vi "UpdateList.vi"(8 "error in (no error)":errorcluster, 11 "Prooduct Actor in":refnum<class "Prooduct Actor.lvclass">) -> (0 "error out":errorcluster, 3 "Prooduct Actor out":refnum<class "Prooduct Actor.lvclass">)   [LabVIEW 2020, in "Prooduct Actor.lvlib" / "Prooduct Actor.lvclass"]
uses:
  Prooduct Actor.lvclass
  Controls/Language Enum.ctl
  Controls/Currency Enum.ctl
  Prooduct Actor.lvclass/Prooduct Actor.ctl
  Read Currency.vi
  Read Language.vi
  Read DBPath.vi
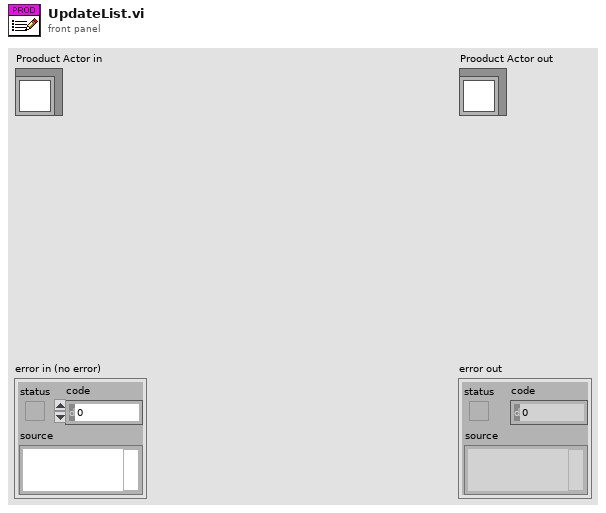
[diagram p1: front panel]
types:
  T1 = typedef "Language Enum.ctl" = enum16{"English", "Español", "Français"}
  T2 = typedef "Currency Enum.ctl" = enum16{"USD", "MXN", "EUR"}
  T3 = cluster{"Language":T1, "Currency":T2, "DB Path":path}
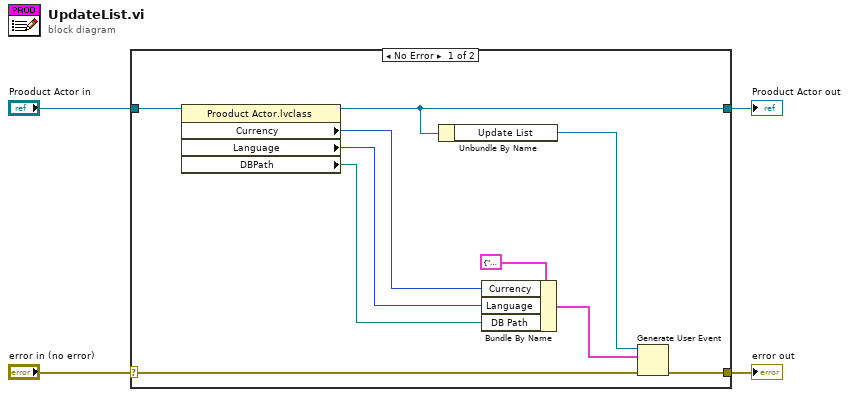
[diagram p0: block diagram]
diagram:
  n1 = case shown="No Error" "error in (no error)" {
    selector: "error in (no error)" -> [w13 w16]
    tunnel: [w12 w16] -> w3
    tunnel: [w11 w15] -> w1
    tunnel: "Prooduct Actor in" -> [w14 w15]
    frame No Error {
      n2 = property class="Prooduct Actor.lvclass"(reference=w14) -> (reference out=w11:refnum<class "Prooduct Actor.lvclass">, "Currency"=w7:T2, "Language"=w6:T1, "DBPath"=w5:path)  [unwired: 1 in, 1 out]
      n3 = Unbundle By Name(w11) -> ("Update List"=w10:refnum<user-event>)
      n4 = Bundle By Name(cluster=T3 {"Language"=enum."English", "Currency"=enum."USD", "DB Path"=path ""} ("event data"), "Currency"=w7, "Language"=w6, "DB Path"=w5) -> (w8:T3)
      n5 = Generate User Event(user event=w10, event data cluster=w8, error in=w13) -> (error out=w12:errorcluster)  [unwired: 1 in, 1 out]
    }
    frame Error {
    }
  }
  "error out" <- w3
  "Prooduct Actor out" <- w1
